vi "Configure Scale Reflection Measurement.vi"(8 "error in (no error)":errorcluster, 9 "Amplitude (0.1 Scale/Division)":dbl=0.1, 10 "Scale Reference Level (0)":dbl, 11 "VISA resource name":refnum<visa-resource-name>) -> (0 "error out":errorcluster, 3 "VISA resource name out":refnum<visa-resource-name>)   [LabVIEW 2022 SP3, in "Agilent N934X Series.lvlib"]
doc: "Configures the Scale settings of reflection measurement mode.\n\nNote:\nThis VI is only applicable for N9321C, N9322C, N9323C, N9324C models."
uses:
  <instrlib>/Agilent N934X Series/Agilent N934X Series.lvlib
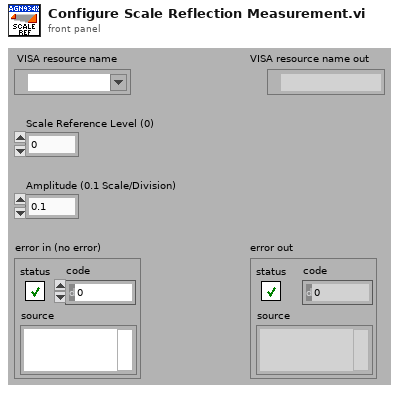
[diagram p1: front panel]
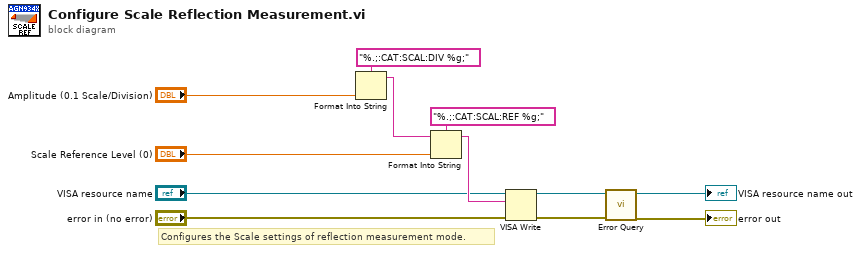
[diagram p0: block diagram]
diagram:
  # "Configures the Scale settings of reflection measurement mode."
  n1 = Format Into String(format string="%.;:CAT:SCAL:DIV %g;", "Amplitude (0.1 Scale/Division)") -> (resulting string=w10:string)  [unwired: 2 in, 1 out]
  n2 = Format Into String(format string="%.;:CAT:SCAL:REF %g;", initial string=w10, "Scale Reference Level (0)") -> (resulting string=w7:string)  [unwired: 1 in, 1 out]
  n3 = VISA Write(VISA resource name="VISA resource name", write buffer=w7, error in (no error)="error in (no error)") -> (VISA resource name out=w4:refnum<visa-resource-name>, error out=w3:errorcluster)  [unwired: 1 out]
  n4 = call <instrlib>:"Error Query.vi"("error in (no error)"=w3, "VISA resource name"=w4) -> ("error out"=→"error out":errorcluster, "VISA resource name out"=→"VISA resource name out":refnum<visa-resource-name>)  [unwired: 6 in, 2 out]
